vi "TStampString.vi"(1 "Incoming string":string, 3 "Previous string":string) -> (0 "String with time stamp":string)   [LabVIEW 2023]
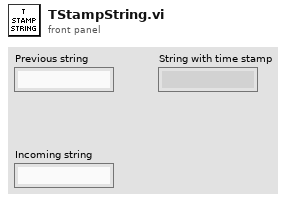
[diagram p1: front panel]
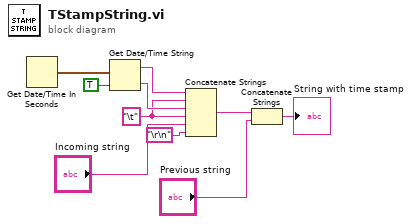
[diagram p0: block diagram]
diagram:
  w8 = "\t" ("string")
  n1 = Get Date/Time In Seconds() -> (seconds since 1Jan1904=w1:timestamp)
  n2 = Get Date/Time String(seconds (now)=w1, want seconds? (F)=TRUE) -> (date string=w10:string, time string=w9:string)  [unwired: 1 in]
  n3 = Concatenate Strings(w10, w8, w9, w8, "Incoming string", "\r\n") -> (w6:string)
  n4 = Concatenate Strings(w6, "Previous string") -> (→"String with time stamp":string)
